vi "Get Symbols Path.vi"() -> (3 "path":path)   [LabVIEW 2020, in "Peek Window.lvlib"]
uses:
  Peek Window.lvlib
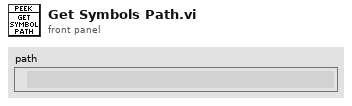
[diagram p1: front panel]
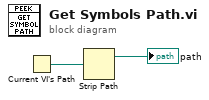
[diagram p0: block diagram]
diagram:
  n1 = Current VI's Path() -> (path=w2:path)
  n2 = Strip Path(path=w2) -> (stripped path=→"path":path)  [unwired: 1 out]
